vi "initialize_instruments (SubVI).vi"(0 "VISA Refnum in":refnum<visa-resource-name>="GPIB0::10::INSTR", 1 "Sample rate":dbl=1000.0 format="%0.2f", 3 "trig_wfm":bool, 5 "Electrode outupt channels":tag="Dev4/ao0", 7 "make volt file":bool, 9 "volt file path":path, 11 "Use synth?":bool, 12 "use arbitrary \nelec waveform?":bool, 13 "elec waveform file":path) -> (4 "instrument config":T1, 6 "Volt vs pos array":cluster{dbl, dbl}[](array[cluster]), 15 "arb electrode arr":dbl[][](array[numeric]))   [LabVIEW 2014]
uses:
  <vilib>/DAQmx/create/channels.llb/DAQmx Create Channel (AO-Voltage-Basic).vi
  <vilib>/DAQmx/configure/timing.llb/DAQmx Timing (Sample Clock).vi
  <vilib>/Utility/file.llb/Read From Spreadsheet File (DBL).vi
  <resource>/objmgr/daqmx.rc
panel:
  out "SampClk.Rate":dbl
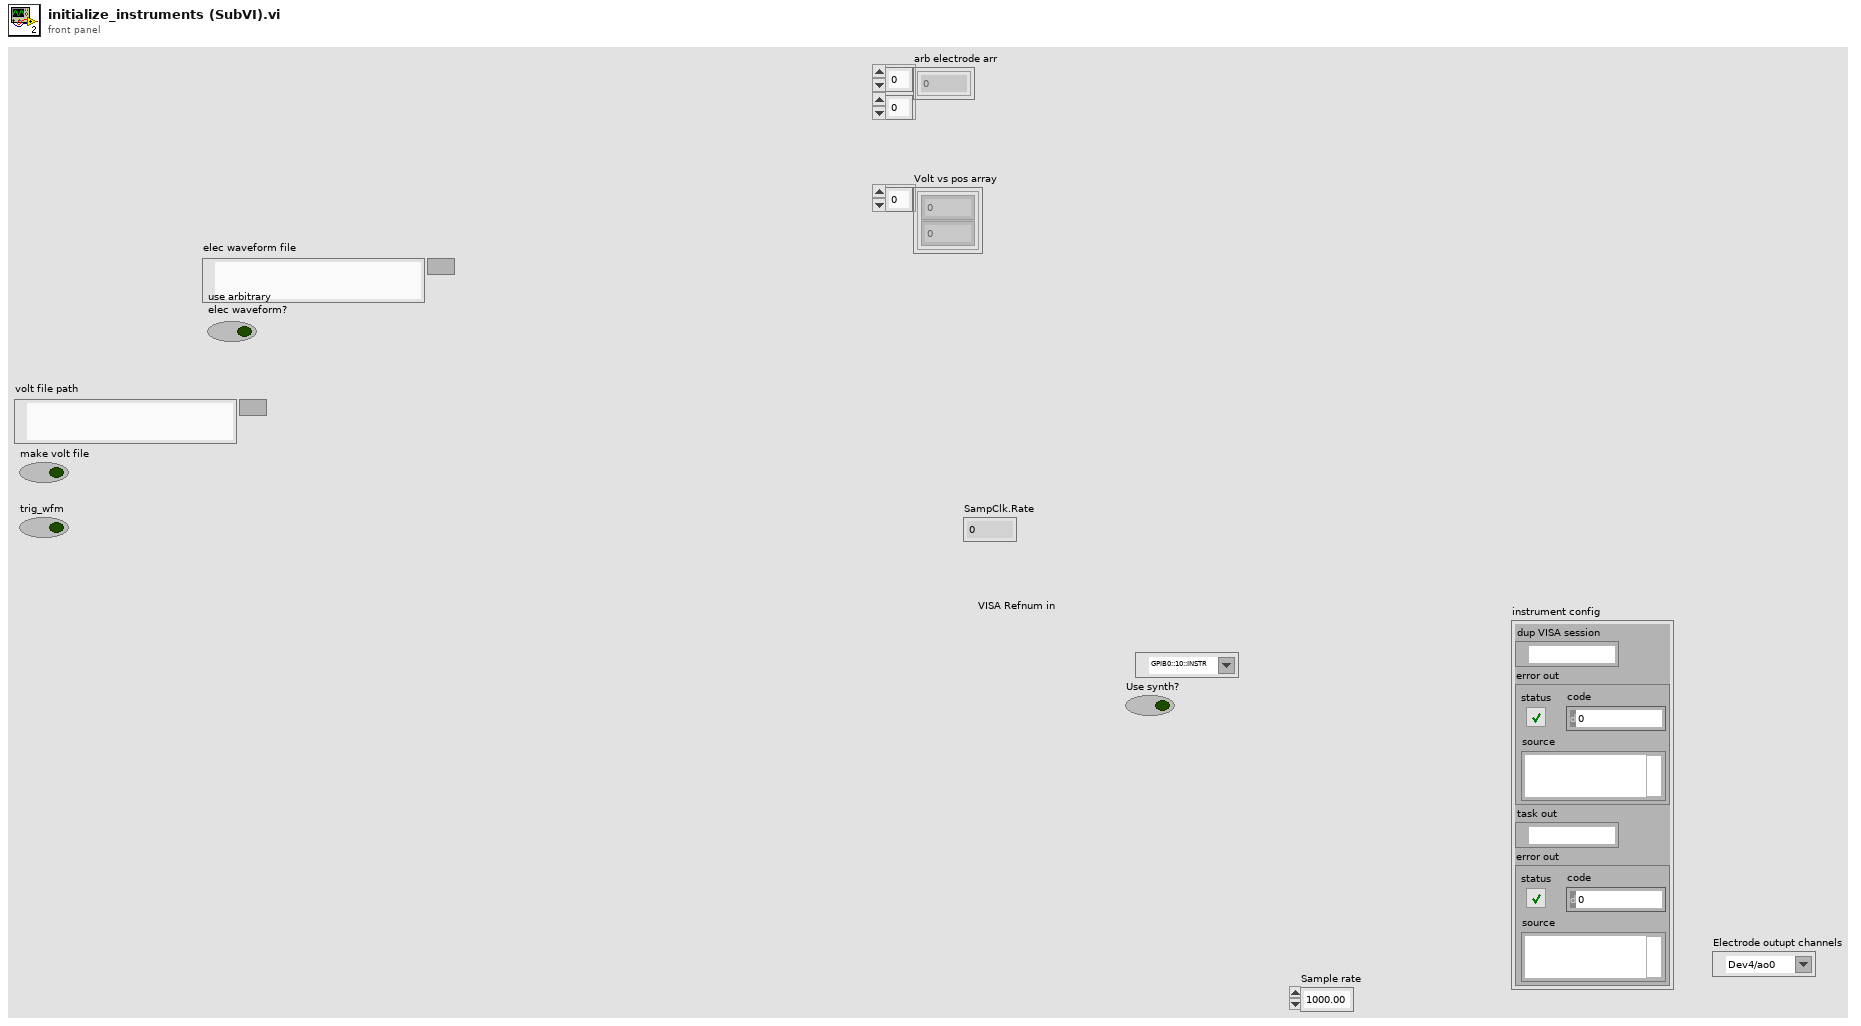
[diagram p1: front panel]
types:
  T1 = cluster{"dup VISA session":refnum<visa-resource-name>, "error out":errorcluster, "task out":refnum<k21>, "error out":errorcluster}
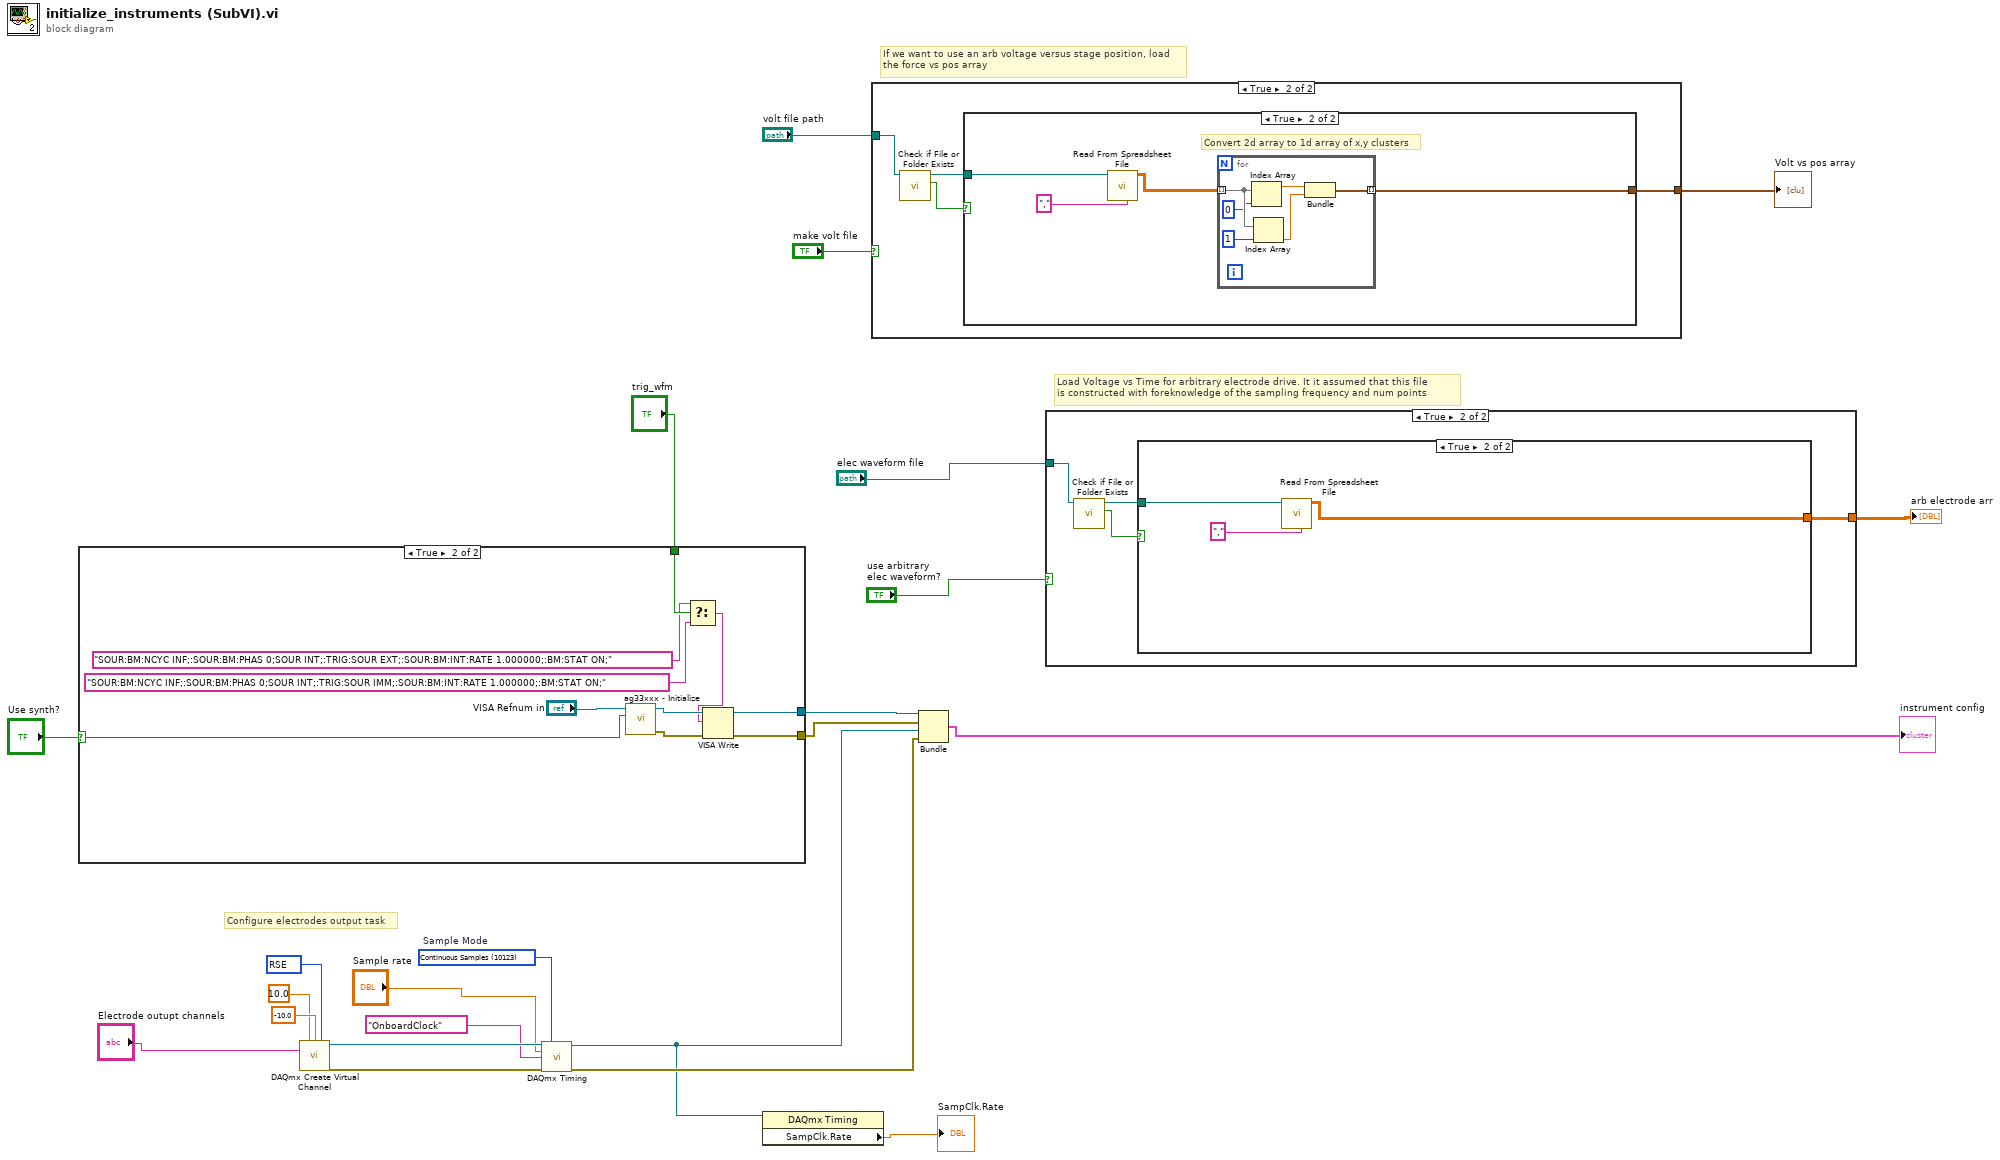
[diagram p0: block diagram]
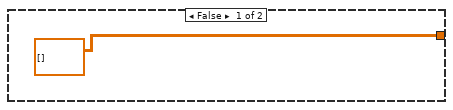
[diagram p2: hidden frame]
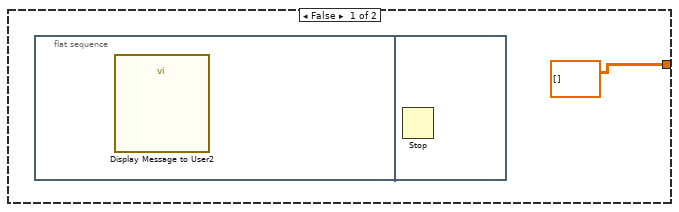
[diagram p3: hidden frame]
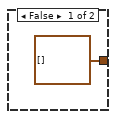
[diagram p4: hidden frame]
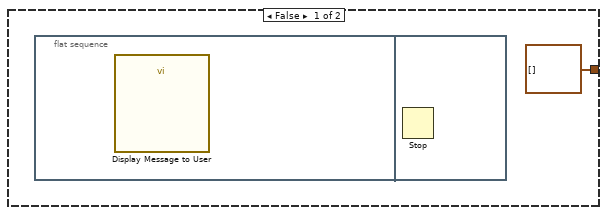
[diagram p5: hidden frame]
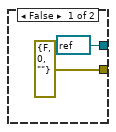
[diagram p6: hidden frame]
diagram:
  w14 = 10083 items=["Default"=-1, "RSE"=10083, "Differential"=10106, "Pseudodifferential"=12529] ("output terminal configuration")
  w20 = 10123 items=["Finite Samples"=10178, "Continuous Samples"=10123, "Hardware Timed Single Point"=12522]  # Sample Mode
  # "Load Voltage vs Time for arbitrary electrode drive. It it assumed that this file\nis constructed with foreknowledge of the sampling frequency and num points"
  # "If we want to use an arb voltage versus stage position, load\nthe force vs pos array"
  # "Configure electrodes output task"
  n1 = case shown="True" "Use synth?" {
    selector: "Use synth?" -> [_ w30]
    tunnel: [refnum<visa-resource-name> refnum ("dup VISA session") w32] -> w22
    tunnel: [errorcluster {"status"=FALSE, "code"=0, "source"=""} ("error out") w31] -> w21
    tunnel: "trig_wfm" -> [_ w29]
    frame False {
    }
    frame True {
      n2 = call "ag33xxx - Initialize.vi"("ID Query (T: Check)"=w30, "Instrument Resource Name"="VISA Refnum in") -> ("error out"=w34:errorcluster, "dup VISA session"=w33:refnum<visa-resource-name>)  [unwired: 8 in]
      n3 = Select(t="SOUR:BM:NCYC INF;:SOUR:BM:PHAS 0;SOUR INT;:TRIG:SOUR EXT;:SOUR:BM:INT:RATE 1.000000;:BM:STAT ON;" ("write buffer"), s=w29, f="SOUR:BM:NCYC INF;:SOUR:BM:PHAS 0;SOUR INT;:TRIG:SOUR IMM;:SOUR:BM:INT:RATE 1.000000;:BM:STAT ON;" ("write buffer")) -> (s? t:f=w26:string)
      n4 = VISA Write(VISA resource name=w33, write buffer=w26, error in (no error)=w34) -> (VISA resource name out=w32:refnum<visa-resource-name>, error out=w31:errorcluster)  [unwired: 1 out]
    }
  }
  n5 = call-poly <vilib>:"DAQmx Create Virtual Channel.vi"("maximum value"=10.0, "minimum value"=-10.0, "output terminal configuration"=w14, "physical channels"="Electrode outupt channels") -> ("task out"=w18:refnum<k21>, "error out"=w19:errorcluster)  [unwired: 10 in]
  n6 = call-poly <vilib>:"DAQmx Timing.vi"("task/channels in"=w18, "sample mode"=w20, "rate"="Sample rate", "source"=tag "OnboardClock" ("Sample Clock Source"), "error in"=w19) -> ("task out"=w10:refnum<k21>, "error out"=w12:errorcluster)  [unwired: 9 in]
  n7 = property class="DAQmx Timing"(reference=w10) -> ("SampClk.Rate"=→"SampClk.Rate":dbl)  [unwired: 1 in, 2 out]
  n8 = case shown="True" "make volt file" {
    tunnel: "volt file path" -> [_ w39]
    tunnel: [cluster{dbl, dbl}[] [] w37] -> w4
    frame False {
    }
    frame True {
      n9 = call <vilib>:"Check if File or Folder Exists.vi"("path"=w39) -> ("file or folder exists?"=w40:bool, "dup path"=w38:path)  [unwired: 8 in, 1 out]
      n10 = case shown="True" w40 {
        tunnel: w38 -> [_ w44]
        tunnel: [cluster{dbl, dbl}[] [] w42] -> w37
        frame False {
          n11 = flat-sequence {
            frame #0 {
              n12 = call "Display Message to User"() -> ()  [unwired: 10 in, 2 out]
            }
            frame #1 {
              n13 = Stop() -> ()  [unwired: 1 in]
            }
          }
        }
        frame True {
          # "Convert 2d array to 1d array of x,y clusters"
          n14 = call-poly <vilib>:"Read From Spreadsheet File.vi"("delimiter (\\t)"="," ("delimiter (\\t)"), "file path (dialog if empty)"=w44) -> ("all rows"=w43:dbl[][])  [unwired: 5 in, 4 out]
          n15 = for {
            tunnel: w43 -> [w51] mode=indexing
            tunnel: [w46] -> w42 mode=indexing
            n16 = Index Array(array=w51, index=0) -> (element=w48:dbl)
            n17 = Index Array(array=w51, index=1) -> (element=w47:dbl)
            n18 = Bundle(w48, w47) -> (w46:cluster{dbl, dbl})  [unwired: 1 in]
          }
        }
      }
    }
  }
  "Volt vs pos array" <- w4
  n19 = Bundle("dup VISA session"=w22, "error out"=w21, "task out"=w10, "error out"=w12) -> (→"instrument config":T1)  [unwired: 1 in]
  n20 = case shown="True" "use arbitrary \nelec waveform?" {
    tunnel: "elec waveform file" -> [_ w55]
    tunnel: [dbl[][] [] ("all rows") w53] -> w1
    frame False {
    }
    frame True {
      n21 = call <vilib>:"Check if File or Folder Exists.vi"("path"=w55) -> ("file or folder exists?"=w56:bool, "dup path"=w54:path)  [unwired: 8 in, 1 out]
      n22 = case shown="True" w56 {
        tunnel: w54 -> [_ w59]
        tunnel: [dbl[][] [] ("all rows") w58] -> w53
        frame False {
          n23 = flat-sequence {
            frame #0 {
              n24 = call "Display Message to User2"() -> ()  [unwired: 10 in, 2 out]
            }
            frame #1 {
              n25 = Stop() -> ()  [unwired: 1 in]
            }
          }
        }
        frame True {
          n26 = call-poly <vilib>:"Read From Spreadsheet File.vi"("delimiter (\\t)"="," ("delimiter (\\t)"), "file path (dialog if empty)"=w59) -> ("all rows"=w58:dbl[][])  [unwired: 5 in, 4 out]
        }
      }
    }
  }
  "arb electrode arr" <- w1
